vi "Write External Payload.vi"(8 "error in (no error)":errorcluster, 9 "Timeout (ms)":i32, 10 "U8 With Header in":u8[](array[numeric]), 11 "CIFFIFO in":refnum<class "CIF_CIPC_Fifo_U8.lvclass">) -> (0 "error out":errorcluster, 1 "timed out?":bool, 2 "U8 With Header out":u8[](array[numeric]), 3 "CIFFIFO out":refnum<class "CIF_CIPC_Fifo_U8.lvclass">)   [LabVIEW 2021, in "CIF_CIPC_Fifo_U8.lvclass"]
uses:
  CIF_CIPC_Fifo_U8.lvclass
  CIF_CIPC_Fifo_U8.lvclass/CIF_CIPC_Fifo_U8.ctl
  CIFChannels/CIFChannels.lvclass
  ChannelCommon/ChannelCommon.lvlib
  ChannelCommon/typedef/TimeStamps.ctl
  D:/dev/Packages/CIF_Channels_Core/src/CIPC_Channels/CIF_CIPC_Chan/CIF_CIPC_Chn.lvclass
  D:/dev/Packages/CIF_Channels_Core/src/CIFChannels/CIFChannels.lvclass
  D:/dev/Packages/CIF_Channels_Core/src/CIPC_Channels/FIFO_U8/CIF_CIPC_Fifo_U8.lvclass
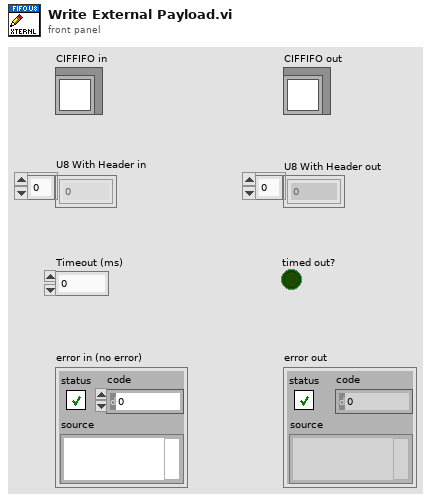
[diagram p1: front panel]
types:
  T1 = typedef "ChannelCommon.lvlib/TimeStamps.ctl" = cluster{"ClockID":u8, "T0":i64, "T_Out":i64}
  T2 = typedef "ChannelCommon.lvlib/FIFO Header.ctl" = cluster{"Length":u64, "T0":i64, "T_Out":i64, "T_Tx":i64, "Ctr":u64, "ClockID":u8}
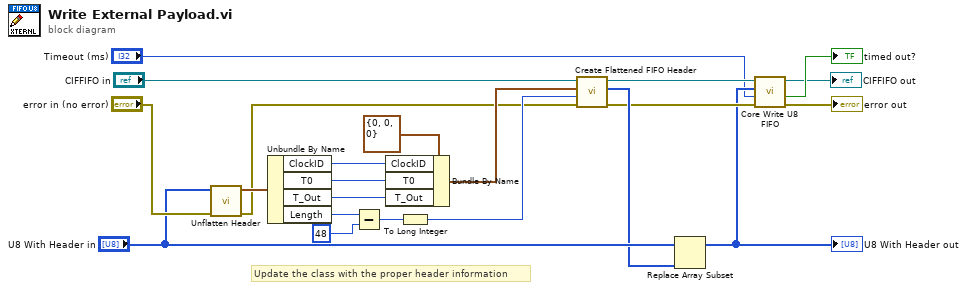
[diagram p0: block diagram]
diagram:
  # "Update the class with the proper header information"
  n1 = call "Unflatten Header.vi"("error in (no error)"="error in (no error)", "Flattened Data in"="U8 With Header in") -> ("error out"=w11:errorcluster, "Header out"=w22:T2)  [unwired: 7 in, 1 out]
  n2 = Unbundle By Name(w22) -> ("ClockID"=w13:u8, "T0"=w14:i64, "T_Out"=w15:i64, "Length"=w21:u64)
  n3 = Subtract(x=w21, y=u64 48) -> (x-y=w19:u64)
  n4 = Bundle By Name(cluster=T1 {"ClockID"=0, "T0"=0, "T_Out"=0} ("FIFO Timestamps"), "ClockID"=w13, "T0"=w14, "T_Out"=w15) -> (w16:T1)
  n5 = To Long Integer(number=w19) -> (32bit integer=w18:i32)
  n6 = call "Create Flattened FIFO Header.vi"("error in (no error)"=w11, "Data Length"=w18, "FIFO Timestamps"=w16, "CIFChannels in"="CIFFIFO in") -> ("error out"=w7:errorcluster, "Flattened FIFO Header"=w9:u8[], "CIFChannels out"=w8:refnum<class "CIF_CIPC_Fifo_U8.lvclass">)  [unwired: 5 in]
  n7 = Replace Array Subset(array="U8 With Header in", new element=w9) -> (w4:u8[])  [unwired: 1 in]
  "U8 With Header out" <- w4
  n8 = call "Core Write U8 FIFO.vi"("error in (no error)"=w7, "Timeout (ms)"="Timeout (ms)", "U8 With Header in"=w4, "CIFFIFO in"=w8) -> ("error out"=→"error out":errorcluster, "timed out?"=→"timed out?":bool, "CIFFIFO out"=→"CIFFIFO out":refnum<class "CIF_CIPC_Fifo_U8.lvclass">)  [unwired: 4 in, 1 out]
